vi "CreateClassesVI.vi"(4 "Factory Class Path":path, 6 "Agents class path":path, 8 "error in":errorcluster, 9 "FactoryFolder":path, 10 "Visitor Class Paths":path[](array[path])) -> (0 "error out":errorcluster, 3 "classesVIPath":path)   [LabVIEW 2009, in "HGF_VisitorGenerator.lvlib"]
doc: "create factory's override classes.vi"
uses:
  HGF_VisitorGenerator.lvlib
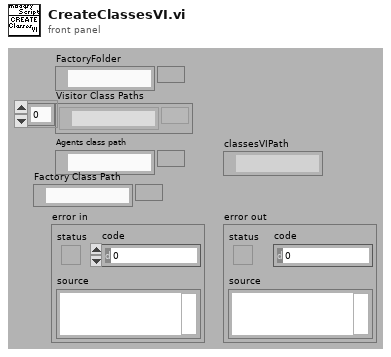
[diagram p1: front panel]
types:
  T1 = enum32{"invalid VI type", "Standard VI", "Control VI", "Global VI", "Polymorphic VI", "Configuration VI", "SubSystem", "Facade VI", "Method VI", "Statechart Diagram VI"}
  T2 = enum16{"Invalid Wire Rule", "Required", "Recommended", "Optional", "Dynamic Dispatch"}
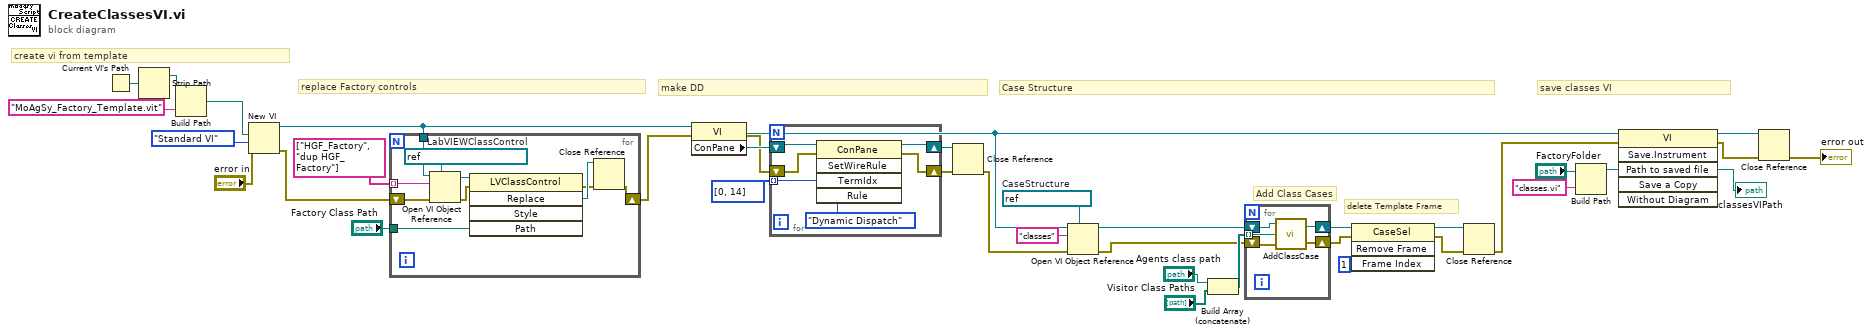
[diagram p0: block diagram]
diagram:
  w22 = refnum<vi> refnum  # CaseStructure
  # "replace Factory controls"
  # "delete Template Frame"
  # "Add Class Cases"
  # "Case Structure"
  # "save classes VI"
  # "make DD"
  # "create vi from template"
  n1 = Current VI's Path() -> (path=w31:path)
  n2 = Strip Path(path=w31) -> (stripped path=w1:path)  [unwired: 1 out]
  n3 = Build Path(base path=w1, name or relative path="MoAgSy_Factory_Template.vit") -> (appended path=w3:path)
  n4 = New VI(8:"error in", 9:T1."Standard VI" ("vi type (standard vi)"), 10:w3) -> (0:w9:errorcluster, 3:w10:refnum<vi>)  [unwired: 4 in]
  n5 = for {
    tunnel: w10 -> [w47]
    tunnel: "Factory Class Path" -> [w43]
    tunnel: string[] ["HGF_Factory", "dup HGF_Factory"] -> [w39] mode=indexing
    shift-right: [w38] -> w6
    shift-left: w9 -> [w45]
    w46 = refnum<vi> refnum  # LabVIEWClassControl
    n6 = Open VI Object Reference(7:w46, 8:w45, 10:w39, 11:w47) -> (0:w42:errorcluster, 3:w44:refnum<vi>)
    n7 = invoke class="LVClassControl" method="Replace"(reference=w44, error in=w42, "Path"=w43) -> (error out=w40:errorcluster, "Replace"=w41:refnum<vi>)  [unwired: 2 in, 3 out]
    n8 = Close Reference(reference=w41, error in (no error)=w40) -> (error out=w38:errorcluster)
  }
  n9 = property class="VI"(reference=w10, error in=w6) -> (reference out=w23:refnum<vi>, error out=w28:errorcluster, "ConPane"=w29:refnum<vi>)
  n10 = for {
    shift-right: [w50] -> w26
    shift-left: w28 -> [w51]
    shift-right: [w49] -> w27
    shift-left: w29 -> [w52]
    tunnel: u32[] [0, 14] -> [w48] mode=indexing
    n11 = invoke class="ConPane" method="SetWireRule"(reference=w52, error in=w51, "TermIdx"=w48, "Rule"=T2."Dynamic Dispatch") -> (reference out=w49:refnum<vi>, error out=w50:errorcluster)  [unwired: 1 in, 3 out]
  }
  n12 = Close Reference(reference=w27, error in (no error)=w26) -> (error out=w20:errorcluster)
  n13 = Open VI Object Reference(7:w22, 8:w20, 10:"classes" ("name/order"), 11:w23) -> (0:w4:errorcluster, 3:w5:refnum<vi>)
  n14 = Build Array (concatenate)("Agents class path", "Visitor Class Paths") -> (w13:path[])
  n15 = for {
    tunnel: w13 -> [w54] mode=indexing
    shift-right: [w57] -> w16
    shift-left: w5 -> [w58]
    shift-right: [w55] -> w15
    shift-left: w4 -> [w56]
    n16 = call "AddClassCase.vi"("error in"=w56, "Class path"=w54, "CaseSel Refnum"=w58) -> ("error out"=w55:errorcluster, "dup CaseSel Refnum"=w57:refnum<vi>)
  }
  n17 = invoke class="CaseSel" method="Remove Frame"(reference=w16, error in=w15, "Frame Index"=u32 1) -> (reference out=w12:refnum<vi>, error out=w11:errorcluster)  [unwired: 1 in, 2 out]
  n18 = Close Reference(reference=w12, error in (no error)=w11) -> (error out=w19:errorcluster)
  n19 = Build Path(base path="FactoryFolder", name or relative path="classes.vi") -> (appended path=w32:path)
  "classesVIPath" <- w32
  n20 = invoke class="VI" method="Save.Instrument"(reference=w23, error in=w19, "Path to saved file"=w32) -> (reference out=w35:refnum<vi>, error out=w34:errorcluster)  [unwired: 3 in, 4 out]
  n21 = Close Reference(reference=w35, error in (no error)=w34) -> (error out=→"error out":errorcluster)
